vi "Write Responder.vi"(8 "error in (no error)":errorcluster, 10 "BaseResponder.lvclass":refnum<class "BaseResponder.lvclass">, 11 "BaseDriver in":refnum<class "BaseDriver.lvclass">) -> (0 "error out":errorcluster, 3 "BaseDriver out":refnum<class "BaseDriver.lvclass">)   [LabVIEW 2013, in "BaseDriver.lvclass"]
doc: "The Responder is the object that will return data from remote destination to the calling application. It should be a child of the BaseResponder class and contains overloadded methods for emitting responses, such as to a queue or an event"
uses:
  BaseDriver.lvclass
  Responder/BaseResponder/BaseResponder.lvclass
  BaseDriver.lvclass/BaseDriver.ctl
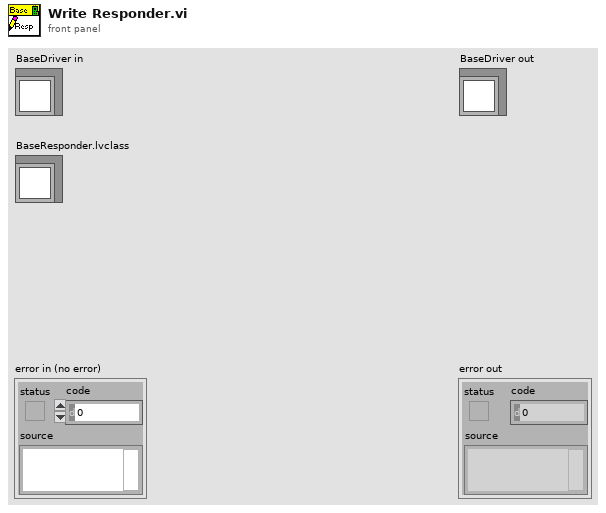
[diagram p1: front panel]
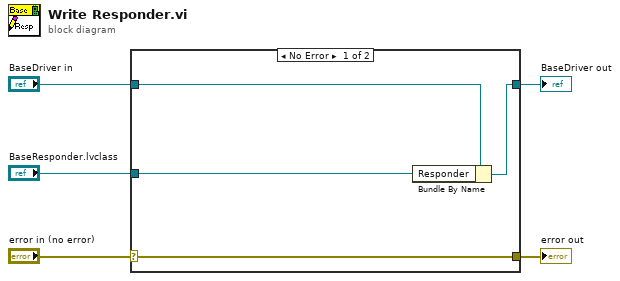
[diagram p0: block diagram]
diagram:
  n1 = case shown="No Error" "error in (no error)" {
    selector: "error in (no error)" -> [w9 w10]
    tunnel: [w9 w10] -> w4
    tunnel: [w7 w11] -> w2
    tunnel: "BaseDriver in" -> [w8 w11]
    tunnel: "BaseResponder.lvclass" -> [w6 _]
    frame No Error {
      n2 = Bundle By Name(cluster=w8, "Responder"=w6) -> (w7:refnum<class "BaseDriver.lvclass">)
    }
    frame Error {
    }
  }
  "error out" <- w4
  "BaseDriver out" <- w2
